vi "CRYGraph Octave Window.vi"() -> ()   [LabVIEW 2013]
uses:
  <vilib>/Utility/miscctls.llb/LVPoint32TypeDef.ctl
  Control/CRYFlag Cluster.ctl
  <vilib>/Utility/miscctls.llb/LVRowAndColumnTypeDef.ctl
  <vilib>/Utility/miscctls.llb/LVRectTypeDef.ctl
  SubVI/CRYData View Global.vi
  SubVI/CRYMain Sub Window Global.vi
  CRYCurveLibrary/Global/CRYCurve Library Global.vi
panel:
  out "LegendVScrollShow":bool=TRUE
  out "Legend Ref":refnum<vi>
  out "SelectedRow":i32[](array[numeric])
  in  "LoadFinish":bool
  in  "ScaleFitY 2":bool
  in  "ScaleFitY":bool
  in  "ScaleFitX":bool
  in  "ToolbarUpdate":bool
  out "PropertyTab":string
  in  "OpenProperty":bool
  in  "PaletteShow":bool
  in  "FitPanes":bool
  in  "DirectionKey":bool
  out "Graph Ref":refnum<vi>
  out "Repaint Watermark":i32
  out "Event Name":string
  out "ReportDrop":bool
  in  "AxisChange":bool
  in  "RemoveSome":bool
  in  "RemoveAll":bool
  in  "CursorColor":bool
  out "NewCursIdx":u32
  out "Test":string
  in  "OldCursIdx":u32
  out "Queue Name":string
  in  "StateOut":bool
  out "Cursor Coords":T1
  in  "CursorPlot":bool
  out "Cursor Ref":refnum<vi>
  in  "CursorShow":bool
  out "Octave Graph":cluster{"XY Graph":cluster{dbl, dbl}[]}[](graph)
  out "Title Name":string
  out "OldRow":i32
  out "TotalPlot":u32
  out "Graph Number":i32
  in  "stop":bool
  in  "CursorEnabled":bool
  in  "Cursor":string[][](table)
  in  "LegendShow":bool
  in  "ColorBox":u32(colorbox)
  in  "Legend":i32[](listbox)
  in  "GraphType":string
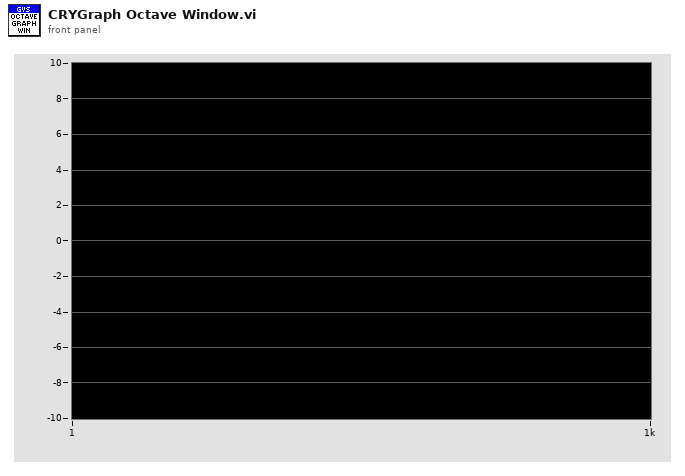
[diagram p1: front panel]
types:
  T1 = typedef "LVPoint32TypeDef.ctl" = cluster{"Horizontal":i32, "Vertical":i32}
  T2 = typedef "CRYFlag Cluster.ctl" = cluster{"LegendShow":bool, "CellClick":bool, "Total Number":bool, "ScaleFitX":bool, "ScaleFitY":bool, "MapModeX":u8, "MapModeY":u8, "CursorShow":bool, "MagnitudeShow":bool, "PreviewShow":bool, "CursorEnabled":bool, "IntensityShow":bool, "PaletteShow":bool, "PhaseShow":bool, "XYShow":bool, "FrequencyShow":bool, "LegendVScrollShow":bool, "FrequencyVScrollShow":bool}
  T3 = typedef "CRYGraph Event.ctl" = cluster{"EvenName":string, "TitleName":string, "GraphName":string, "GraphType":string, "Data":variant, "Queue Name":string, "DataView Number":i32}
  T4 = enum16{"No Scaling", "Scale All Objects", "Scale Single Object"}
  T5 = typedef "LVRowAndColumnTypeDef.ctl" = cluster{"Row":i32, "Column":i32}
  T6 = typedef "LVRectTypeDef.ctl" = cluster{"Left":i16, "Top":i16, "Right":i16, "Bottom":i16}
  T7 = typedef "LVBoundsTypeDef.ctl" = cluster{"Width":u32, "Height":u32}
  T8 = typedef "LVPositionTypeDef.ctl" = cluster{"Left":i32, "Top":i32}
  T9 = typedef "CRYData Cluster.ctl" = cluster{"Name":string, "Curve":cluster{"x":dbl, "y":dbl, "z":dbl}[], "X data":u16, "Y data":u16, "Z data":u16, "X axis":u16, "Y axis":u16, "Z axis":u16, "X unit":string, "Y unit":string, "Z unit":string, "X dB ref":dbl, "Y dB ref":dbl, "Z dB ref":dbl, "single val":bool, "protected":bool, "display X":bool, "display Y":bool, "display Z":bool, "Test Info":string, "Step No.":i32, "Plot Settings":cluster{"Color":u32, "Interpolation":u8, "Point Style":u8, "Line Style":u8, "Point Color":u32, "Line Width":u8, "Bar Plot Style":u8, "Fill To":i16}, "AutoProtect":bool}
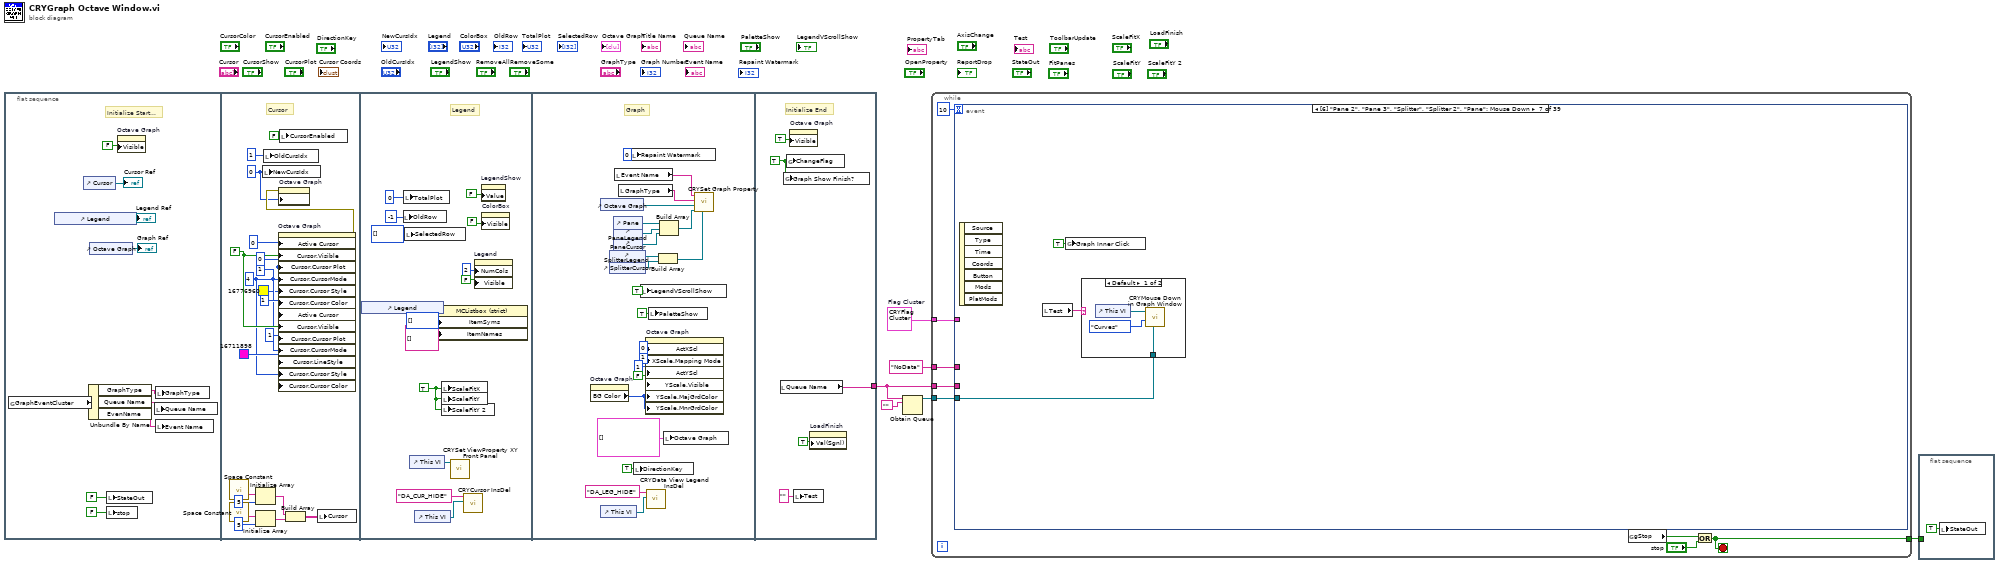
[diagram p0: block diagram]
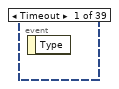
[diagram p2: hidden frame]
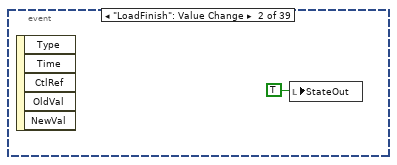
[diagram p3: hidden frame]
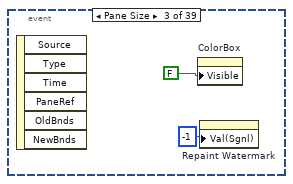
[diagram p4: hidden frame]
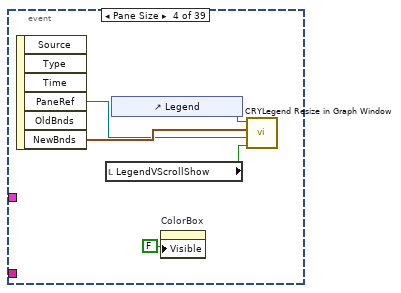
[diagram p5: hidden frame]
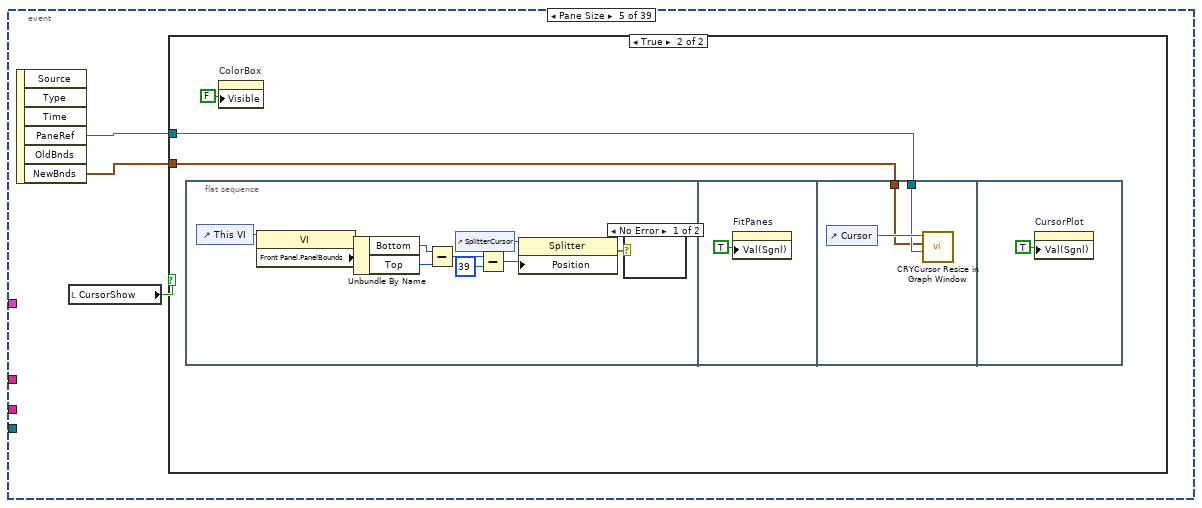
[diagram p6: hidden frame]
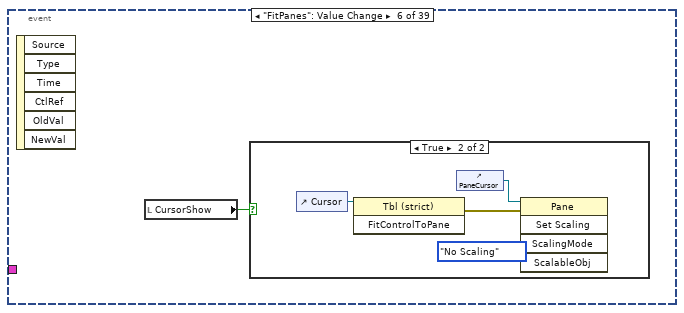
[diagram p9: hidden frame]
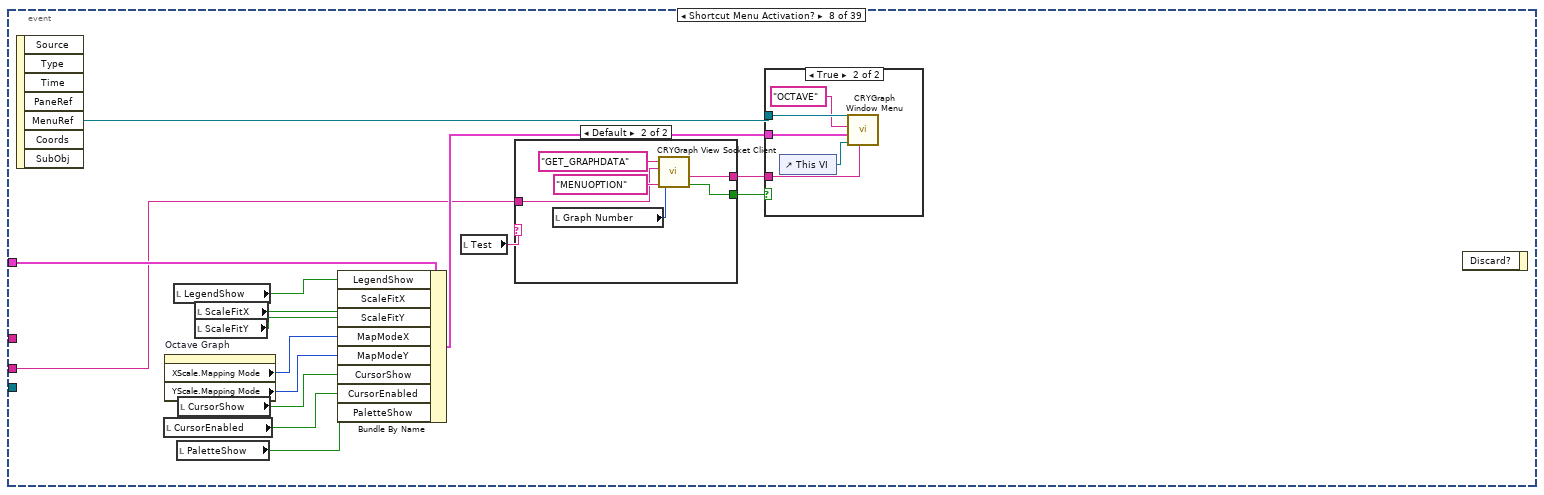
[diagram p12: hidden frame]
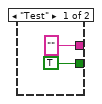
[diagram p13: hidden frame]
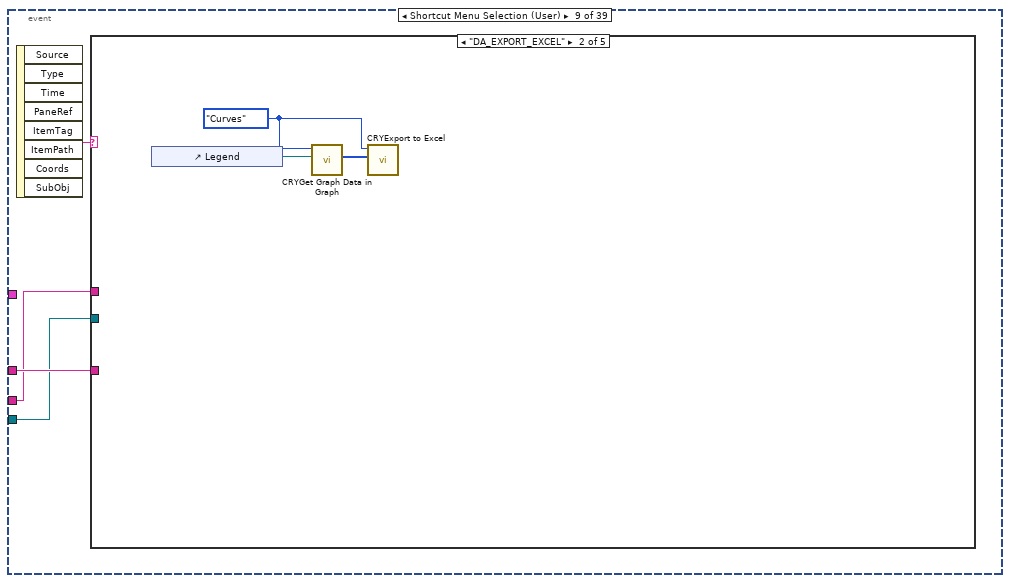
[diagram p15: hidden frame]
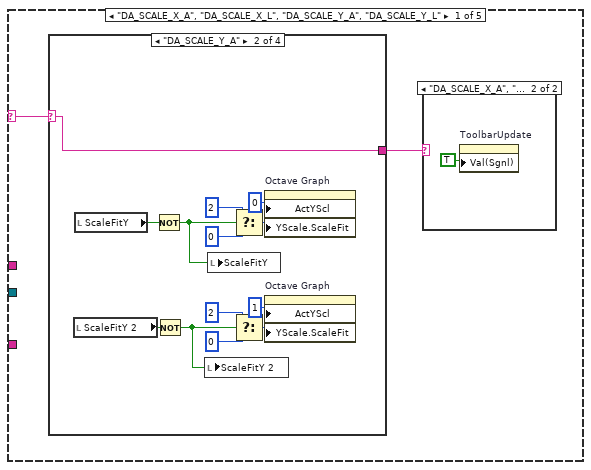
[diagram p16: hidden frame]
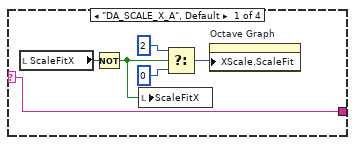
[diagram p18: hidden frame]
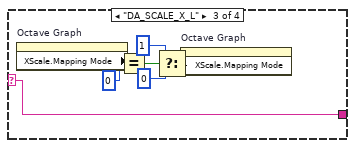
[diagram p19: hidden frame]
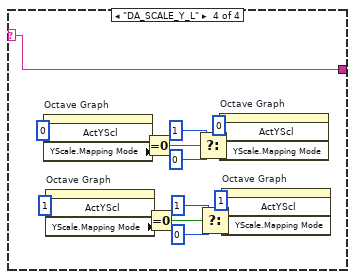
[diagram p20: hidden frame]
diagram:
  w4 = T2 {"LegendShow"=FALSE, "CellClick"=FALSE, "Total Number"=FALSE, "ScaleFitX"=FALSE, "ScaleFitY"=FALSE, "MapModeX"=0, "MapModeY"=0, "CursorShow"=FALSE, "MagnitudeShow"=FALSE, "PreviewShow"=FALSE, "CursorEnabled"=FALSE, "IntensityShow"=FALSE, "PaletteShow"=FALSE, "PhaseShow"=FALSE, "XYShow"=FALSE, "FrequencyShow"=FALSE, "LegendVScrollShow"=FALSE, "FrequencyVScrollShow"=FALSE}  # Flag Cluster
  n1 = flat-sequence {
    tunnel: [w74] -> w2
    frame #0 {
      # "Initialize Start..."
      n2 = global read "CRYData View Global.vi" "GraphEventCluster"() -> (w12:T3)
      n3 = control-ref of="Legend"() -> (→"Legend Ref":refnum<vi>)
      n4 = control-ref of="Cursor"() -> (→"Cursor Ref":refnum<vi>)
      n5 = Unbundle By Name(w12) -> ("GraphType"=w10:string, "Queue Name"=w11:string, "EvenName"=w9:string)
      n6 = control-ref of="Octave Graph"() -> (→"Graph Ref":refnum<vi>)
      n7 = local write "StateOut"(FALSE ("StateOut")) -> ()
      n8 = local write "stop"(FALSE ("stop")) -> ()
      n9 = property on="Octave Graph" class="XYGraph (strict)"("Visible"=FALSE) -> ()  [unwired: 2 in, 2 out]
      n10 = local write "Queue Name"(w11) -> ()
      n11 = local write "GraphType"(w10) -> ()
      n12 = local write "Event Name"(w9) -> ()
    }
    frame #1 {
      w22 = u32 0 ("Active Cursor")
      w17 = u8 4 ("Cursor.Cursor Style")
      w24 = u32 1 ("Cursor.Cursor Mode")
      w25 = 0 ("Cursor.Cursor Plot")
      w26 = FALSE ("Cursor.Visible")
      # "Cursor"
      n13 = call <vilib>:"Space Constant.vi"() -> ("String"=w30:string)
      n14 = call <vilib>:"Space Constant.vi"() -> ("String"=w35:string)
      n15 = Initialize Array(w30, 5 ("dimension size")) -> (w32:string[])
      n16 = Initialize Array(w35, 5 ("dimension size")) -> (w36:string[])
      n17 = local write "NewCursIdx"(w22) -> ()
      n18 = local write "OldCursIdx"(u32 1 ("OldCursIdx")) -> ()
      n19 = property on="Octave Graph" class="XYGraph (strict)"("Active Cursor"=u32 0, "Cursor.Visible"=w26, "Cursor.Cursor Plot"=w25, "Cursor.CursorMode"=w24, "Cursor.Cursor Style"=w17, "Cursor.Cursor Color"=u32 16776960, "Active Cursor"=u32 1, "Cursor.Visible"=w26, "Cursor.Cursor Plot"=w25, "Cursor.CursorMode"=w24, "Cursor.LineStyle"=u8 1 ("Cursor.Line Style"), "Cursor.Cursor Style"=w17, "Cursor.Cursor Color"=u32 16711898) -> (error out=w23:errorcluster)  [unwired: 2 in, 1 out]
      n20 = property on="Octave Graph" class="XYGraph (strict)"(error in=w23, "Active Cursor"=w22) -> ()  [unwired: 1 in, 2 out]
      n21 = local write "CursorEnabled"(FALSE ("CursorEnabled")) -> ()
      n22 = Build Array(w32, w36) -> (w33:string[][])
      n23 = local write "Cursor"(w33) -> ()
    }
    frame #2 {
      w38 = TRUE ("ScaleFitX")
      # "Legend"
      n24 = control-ref of="Legend"() -> (w50:refnum<vi>)
      n25 = local write "OldRow"(-1 ("OldRow 2")) -> ()
      n26 = local write "TotalPlot"(u32 0 ("TotalPlot")) -> ()
      n27 = local write "SelectedRow"(i32[] [] ("SelectedRow")) -> ()
      n28 = control-ref of="This VI"() -> (w39:refnum<vi>)
      n29 = control-ref of="This VI"() -> (w41:refnum<vi>)
      n30 = property on="Property Node" class="MCListbox (strict)"(reference=w50, "ItemSyms"=i32[] [] ("Item Symbols"), "ItemNames"=string[][] [] ("Item Names")) -> ()  [unwired: 1 in, 2 out]
      n31 = local write "ScaleFitX"(w38) -> ()
      n32 = local write "ScaleFitY"(w38) -> ()
      n33 = local write "ScaleFitY 2"(w38) -> ()
      n34 = call "CRYSet ViewProperty XY  Front Panel.vi"("Vi Ref"=w39) -> ()  [unwired: 11 in]
      n35 = call "CRYCursor InsDel.vi"("Graph VI Ref"=w41, "sAction"="DA_CUR_HIDE" ("Action Type")) -> ()  [unwired: 10 in]
      n36 = property on="Legend" class="MCListbox (strict)"("NumCols"=u32 2 ("Number of Columns"), "Visible"=FALSE) -> ()  [unwired: 2 in, 2 out]
      n37 = property on="LegendShow" class="Bool (strict)"("Value"=FALSE ("Visible")) -> ()  [unwired: 2 in, 2 out]
      n38 = property on="ColorBox" class="ColBox"("Visible"=FALSE) -> ()  [unwired: 2 in, 2 out]
    }
    frame #3 {
      # "Graph"
      n39 = property on="Octave Graph" class="XYGraph (strict)"() -> ("BG Color"=w70:u32)  [unwired: 2 in, 2 out]
      n40 = control-ref of="Octave Graph"() -> (w60:refnum<vi>)
      n41 = control-ref of="This VI"() -> (w52:refnum<vi>)
      n42 = control-ref of="SplitterLegend"() -> (w69:refnum<vi>)
      n43 = control-ref of="SplitterCursor"() -> (w68:refnum<vi>)
      n44 = control-ref of="Pane"() -> (w66:refnum<vi>)
      n45 = control-ref of="PaneLegend"() -> (w67:refnum<vi>)
      n46 = control-ref of="PaneCursor"() -> (w55:refnum<vi>)
      n47 = local read "Event Name"() -> (w62:string)
      n48 = local read "GraphType"() -> (w63:string)
      n49 = local write "Repaint Watermark"(0 ("Repaint Watermark")) -> ()
      n50 = local write "DirectionKey"(TRUE ("DirectionKey")) -> ()
      n51 = local write "LegendVScrollShow"(TRUE ("LegendVScrollShow")) -> ()
      n52 = property on="Octave Graph" class="XYGraph (strict)"("ActXScl"=0 ("Active X Scale"), "XScale.Mapping Mode"=u8 1 ("X Scale.Mapping Mode"), "ActYScl"=1 ("Active Y Scale"), "YScale.Visible"=FALSE ("Y Scale.Visible"), "YScale.MajGrdColor"=w70, "YScale.MnrGrdColor"=w70) -> ()  [unwired: 2 in, 2 out]
      n53 = call "CRYData View Legend InsDel.vi"("Graph VI Ref"=w52, "sAction"="DA_LEG_HIDE" ("Action Type")) -> ()  [unwired: 2 in, 8 out]
      n54 = local write "PaletteShow"(TRUE ("PaletteShow")) -> ()
      n55 = Build Array(w69, w68) -> (w64:refnum<vi>[])
      n56 = Build Array(w66, w67, w55) -> (w65:refnum<vi>[])
      n57 = local write "Octave Graph"(cluster{"XY Graph":cluster{dbl, dbl}[]}[] [] ("XY Graph")) -> ()
      n58 = call "CRYSet Graph Property.vi"("Splitters"=w64, "Panes"=w65, "Graph Ref"=w60, "Graph Type"=w63, "Event Name"=w62) -> ()  [unwired: 7 in]
    }
    frame #4 {
      w77 = TRUE ("ChangeFlag")
      # "Initialize End"
      n59 = local read "Queue Name"() -> (w74:string)
      n60 = global write "CRYData View Global.vi" "Graph Show Finish?"(w77) -> ()
      n61 = global write "CRYData View Global.vi" "ChangeFlag"(w77) -> ()
      n62 = property on="Octave Graph" class="XYGraph (strict)"("Visible"=TRUE) -> ()  [unwired: 2 in, 2 out]
      n63 = local write "Test"("" ("Test")) -> ()
      n64 = property on="LoadFinish" class="Bool (strict)"("Val(Sgnl)"=TRUE ("Value (Signaling)")) -> ()  [unwired: 2 in, 2 out]
    }
  }
  n65 = Obtain Queue(name (unnamed)=w2, element data type="") -> (queue out=w6:refnum<queue>)  [unwired: 3 in, 2 out]
  n66 = while {
    tunnel: w6 -> [w85]
    tunnel: w4 -> [w83]
    tunnel: "NoData" ("input 2") -> [w80]
    tunnel: w2 -> [w79]
    tunnel: [w78] -> w1
    stop <- w78 stop-if-true
    n67 = event shown="[6] \"Pane 2\", \"Pane 3\", \"Splitter\", \"Splitter 2\", \"Pane\": Mouse Down" {
      selector: _ -> [_ _ _ _ _ _ _ _ _ _ _ _ _ _ _ _ _ _ _ _ _ _ _ _ _ _ _ _ _ _ _ _ _ _ _ _ _ _ _]
      dyn-events: _ -> [_ _ _ _ _ _ _ _ _ _ _ _ _ _ _ _ _ _ _ _ _ _ _ _ _ _ _ _ _ _ _ _ _ _ _ _ _ _ _]
      timeout: 10 -> [_ _ _ _ _ _ _ _ _ _ _ _ _ _ _ _ _ _ _ _ _ _ _ _ _ _ _ _ _ _ _ _ _ _ _ _ _ _ _]
      tunnel: w85 -> [_ _ _ _ _ _ w121 _ w153 _ w265 _ w318 _ _ _ _ _ _ _ _ _ _ _ _ w525 _ _ _ _ _ w731 _ _ w743 _ _ _ _]
      tunnel: w83 -> [_ _ _ _ _ _ _ w137 _ w242 _ w303 _ _ _ _ _ _ _ _ _ _ _ _ _ _ _ _ _ _ _ _ _ _ _ _ _ _ _]
      tunnel: w80 -> [_ _ _ _ _ _ _ _ w155 _ w262 _ w317 _ _ _ _ _ _ _ _ _ _ _ _ _ _ _ _ _ _ _ _ _ _ _ _ _ _]
      tunnel: w79 -> [_ _ _ _ _ _ _ w131 w154 _ _ _ _ _ _ _ _ _ _ _ _ _ _ _ _ _ _ _ _ _ _ _ _ _ _ _ _ _ _]
      event Timeout {
        n68 = event-data() -> ()  [unwired: 2 out]
      }
      event "LoadFinish": Value Change {
        n69 = event-data() -> ()  [unwired: 6 out]
        n70 = local write "StateOut"(TRUE ("StateOut")) -> ()
      }
      event Pane Size {
        n71 = event-data() -> ()  [unwired: 7 out]
        n72 = property on="ColorBox" class="ColBox"("Visible"=FALSE) -> ()  [unwired: 2 in, 2 out]
        n73 = property on="Repaint Watermark" class="DigNum (strict)"("Val(Sgnl)"=-1 ("Value (Signaling)")) -> ()  [unwired: 2 in, 2 out]
      }
      event Pane Size {
        n74 = event-data() -> ("PaneRef"=w90:refnum<vi>, "NewBnds"=w92:T6)  [unwired: 5 out]
        n75 = local read "LegendVScrollShow"() -> (w89:bool)
        n76 = control-ref of="Legend"() -> (w91:refnum<vi>)
        n77 = property on="ColorBox" class="ColBox"("Visible"=FALSE) -> ()  [unwired: 2 in, 2 out]
        n78 = call "CRYLegend Resize in Graph Window.vi"("VScrollShow"=w89, "Pane Ref"=w90, "input cluster"=w92, "Legend"=w91) -> ()  [unwired: 8 out]
      }
      event Pane Size {
        n79 = event-data() -> ("PaneRef"=w95:refnum<vi>, "NewBnds"=w94:T6)  [unwired: 5 out]
        n80 = local read "CursorShow"() -> (w96:bool)
        n81 = case shown="True" w96 {
          tunnel: w95 -> [_ w98]
          tunnel: w94 -> [_ w97]
          frame False {
          }
          frame True {
            n82 = flat-sequence {
              tunnel: w98 -> [w111]
              tunnel: w97 -> [w110]
              frame #0 {
                n83 = control-ref of="This VI"() -> (w103:refnum<vi>)
                n84 = property class="VI"(reference=w103) -> ("Front Panel.PanelBounds"=w104:T6)  [unwired: 1 in, 2 out]
                n85 = Unbundle By Name(w104) -> ("Bottom"=w101:i16, "Top"=w102:i16)
                n86 = Subtract(x=w101, y=w102) -> (x-y=w105:i16)
                n87 = control-ref of="SplitterCursor"() -> (w108:refnum<vi>)
                n88 = Subtract(x=w105, y=39) -> (x-y=w100:i32)
                n89 = property class="Splitter"(reference=w108, "Position"=w100) -> (error out=w107:errorcluster)  [unwired: 1 in, 1 out]
                n90 = case shown="No Error" w107 {
                  frame No Error {
                  }
                  frame Error {
                  }
                }
              }
              frame #1 {
                n91 = property on="FitPanes" class="Bool (strict)"("Val(Sgnl)"=TRUE ("Value (Signaling)")) -> ()  [unwired: 2 in, 2 out]
              }
              frame #2 {
                n92 = control-ref of="Cursor"() -> (w112:refnum<vi>)
                n93 = call "CRYCursor Resize in Graph Window.vi"("Pane Ref"=w111, "input cluster"=w110, "Graph Cursor Ref"=w112) -> ()  [unwired: 9 in]
              }
              frame #3 {
                n94 = property on="CursorPlot" class="Bool (strict)"("Val(Sgnl)"=TRUE ("Value (Signaling)")) -> ()  [unwired: 2 in, 2 out]
              }
            }
            n95 = property on="ColorBox" class="ColBox"("Visible"=FALSE) -> ()  [unwired: 2 in, 2 out]
          }
        }
      }
      event "FitPanes": Value Change {
        n96 = event-data() -> ()  [unwired: 7 out]
        n97 = local read "CursorShow"() -> (w114:bool)
        n98 = case shown="True" w114 {
          frame False {
          }
          frame True {
            n99 = control-ref of="Cursor"() -> (w118:refnum<vi>)
            n100 = invoke class="Tbl (strict)" method="FitControlToPane"(reference=w118) -> (error out=w117:errorcluster)  [unwired: 2 in, 2 out]
            n101 = control-ref of="PaneCursor"() -> (w115:refnum<vi>)
            n102 = invoke class="Pane" method="Set Scaling"(reference=w115, error in=w117, "ScalingMode"=T4."No Scaling" ("Scaling Mode")) -> ()  [unwired: 2 in, 5 out]
          }
        }
      }
      event Mouse Down {
        n103 = event-data() -> ()  [unwired: 8 out]
        n104 = local read "Test"() -> (w120:string)
        n105 = global write "CRYCurve Library Global.vi" "Graph Inner Click"(TRUE ("Graph Inner Click")) -> ()
        n106 = case shown="Default" w120 {
          tunnel: w121 -> [w124 _]
          frame Default {
            n107 = control-ref of="This VI"() -> (w122:refnum<vi>)
            n108 = call "CRYMouse Down in Graph Window.vi"("Queue"=w124, "Selected Type"=enum16{"Curves", "Values", "Results", "WFM"}."Curves" ("Type"), "pGraph VI In"=w122) -> ()  [unwired: 3 in, 6 out]
          }
          frame "Test" {
          }
        }
      }
      event Shortcut Menu Activation? {
        n109 = event-data() -> ("MenuRef"=w139:refnum<k9>)  [unwired: 7 out]
        n110 = local read "CursorEnabled"() -> (w132:bool)
        n111 = property on="Octave Graph" class="XYGraph (strict)"() -> ("XScale.Mapping Mode"=w135:u8, "YScale.Mapping Mode"=w134:u8)  [unwired: 2 in, 2 out]
        n112 = local read "LegendShow"() -> (w138:bool)
        n113 = local read "PaletteShow"() -> (w127:bool)
        n114 = local read "CursorShow"() -> (w133:bool)
        n115 = local read "ScaleFitX"() -> (w126:bool)
        n116 = local read "ScaleFitY"() -> (w125:bool)
        n117 = Bundle By Name(cluster=w137, "LegendShow"=w138, "ScaleFitX"=w126, "ScaleFitY"=w125, "MapModeX"=w135, "MapModeY"=w134, "CursorShow"=w133, "CursorEnabled"=w132, "PaletteShow"=w127) -> (w136:T2)
        n118 = local read "Test"() -> (w128:string)
        n119 = case shown="Default" w128 {
          tunnel: w131 -> [_ w145]
          tunnel: ["" ("sData Out") w144] -> w130
          tunnel: [TRUE ("bResult Out") w143] -> w129
          frame "Test" {
          }
          frame Default {
            n120 = local read "Graph Number"() -> (w142:i32)
            n121 = call "CRYGraph View Socket Client.vi"("sOption"="MENUOPTION", "nData"=w142, "sData"=w145, "sAction"="GET_GRAPHDATA") -> ("bResult Out"=w143:bool, "sData Out"=w144:string)  [unwired: 4 in, 2 out]
          }
        }
        n122 = case shown="True" w129 {
          tunnel: w139 -> [_ w152]
          tunnel: w136 -> [_ w150]
          tunnel: w130 -> [_ w149]
          frame False {
          }
          frame True {
            n123 = control-ref of="This VI"() -> (w148:refnum<vi>)
            n124 = call "CRYGraph Window Menu.vi"("MenuOption"=w149, "pGraph VI"=w148, "Flag Cluster"=w150, "Type"="OCTAVE", "Runtime Menu Ref In"=w152) -> ()  [unwired: 7 out]
          }
        }
        n125 = event-data() -> ()  [unwired: 2 in, 1 out]
      }
      event Shortcut Menu Selection (User) {
        n126 = event-data() -> ("ItemTag"=w156:string)  [unwired: 8 out]
        n127 = case shown="\"DA_EXPORT_EXCEL\"" w156 {
          selector: w156 -> [w158 _ w205 w238 _]
          tunnel: w155 -> [_ _ w208 _ _]
          tunnel: w154 -> [_ _ _ _ _]
          tunnel: w153 -> [_ _ w206 _ _]
          frame "DA_SCALE_X_A", "DA_SCALE_X_L", "DA_SCALE_Y_A", "DA_SCALE_Y_L" {
            n128 = case shown="\"DA_SCALE_Y_A\"" w158 {
              selector: w158 -> [w162 w175 w179 w200]
              tunnel: [w162 w175 w179 w200] -> w157
              frame "DA_SCALE_X_A", Default {
                n129 = local read "ScaleFitX"() -> (w161:bool)
                n130 = Not(x=w161) -> (.not. x?=w160:bool)
                n131 = local write "ScaleFitX"(w160) -> ()
                n132 = Select(t=u8 2, s=w160, f=u8 0) -> (s? t:f=w163:u8)
                n133 = property on="Octave Graph" class="XYGraph (strict)"("XScale.ScaleFit"=w163) -> ()  [unwired: 2 in, 2 out]
              }
              frame "DA_SCALE_Y_A" {
                n134 = local read "ScaleFitY 2"() -> (w168:bool)
                n135 = local read "ScaleFitY"() -> (w169:bool)
                n136 = Not(x=w169) -> (.not. x?=w167:bool)
                n137 = Not(x=w168) -> (.not. x?=w166:bool)
                n138 = local write "ScaleFitY 2"(w166) -> ()
                n139 = local write "ScaleFitY"(w167) -> ()
                n140 = Select(t=u8 2, s=w167, f=u8 0) -> (s? t:f=w176:u8)
                n141 = Select(t=u8 2, s=w166, f=u8 0) -> (s? t:f=w172:u8)
                n142 = property on="Octave Graph" class="XYGraph (strict)"("ActYScl"=0 ("Active Y Scale"), "YScale.ScaleFit"=w176) -> ()  [unwired: 2 in, 2 out]
                n143 = property on="Octave Graph" class="XYGraph (strict)"("ActYScl"=1 ("Active Y Scale"), "YScale.ScaleFit"=w172) -> ()  [unwired: 2 in, 2 out]
              }
              frame "DA_SCALE_X_L" {
                n144 = property on="Octave Graph" class="XYGraph (strict)"() -> ("XScale.Mapping Mode"=w180:u8)  [unwired: 2 in, 2 out]
                n145 = Equal?(x=w180, y=u8 0) -> (x = y?=w185:bool)
                n146 = Select(t=u8 1, s=w185, f=u8 0) -> (s? t:f=w181:u8)
                n147 = property on="Octave Graph" class="XYGraph (strict)"("XScale.Mapping Mode"=w181) -> ()  [unwired: 2 in, 2 out]
              }
              frame "DA_SCALE_Y_L" {
                n148 = property on="Octave Graph" class="XYGraph (strict)"("ActYScl"=0 ("Active Y Scale")) -> ("YScale.Mapping Mode"=w196:u8)  [unwired: 2 in, 2 out]
                n149 = property on="Octave Graph" class="XYGraph (strict)"("ActYScl"=1 ("Active Y Scale")) -> ("YScale.Mapping Mode"=w189:u8)  [unwired: 2 in, 2 out]
                n150 = Equal To 0?(x=w196) -> (x = 0?=w193:bool)
                n151 = Equal To 0?(x=w189) -> (x = 0?=w192:bool)
                n152 = Select(t=u8 1, s=w193, f=u8 0) -> (s? t:f=w197:u8)
                n153 = Select(t=u8 1, s=w192, f=u8 0) -> (s? t:f=w188:u8)
                n154 = property on="Octave Graph" class="XYGraph (strict)"("ActYScl"=0 ("Active Y Scale"), "YScale.Mapping Mode"=w197) -> ()  [unwired: 2 in, 2 out]
                n155 = property on="Octave Graph" class="XYGraph (strict)"("ActYScl"=1 ("Active Y Scale"), "YScale.Mapping Mode"=w188) -> ()  [unwired: 2 in, 2 out]
              }
            }
            n156 = case shown="\"DA_SCALE_X_A\", \"DA_SCALE_Y_A\"" w157 {
              frame Default {
              }
              frame "DA_SCALE_X_A", "DA_SCALE_Y_A" {
                n157 = property on="ToolbarUpdate" class="Bool (strict)"("Val(Sgnl)"=TRUE ("Value (Signaling)")) -> ()  [unwired: 2 in, 2 out]
              }
            }
          }
          frame "DA_EXPORT_EXCEL" {
            w202 = enum16{"Curves", "Values", "Results", "WFM"}."Curves" ("Type")
            n158 = control-ref of="Legend"() -> (w201:refnum<vi>)
            n159 = call "CRYGet Graph Data in Graph.vi"("Legend Refnum"=w201, "Type In"=w202) -> ("Rows"=w203:i32[])  [unwired: 2 in, 7 out]
            n160 = call "CRYExport to Excel.vi"("Rows"=w203, "Type"=w202) -> ()  [unwired: 2 in, 8 out]
          }
          frame Default {
            n161 = Search/Split String(string=w205, search string/char (-)="#") -> (substring before match=w204:string, match + rest of string=w211:string)  [unwired: 2 out]
            n162 = call "CRYPreUpdate Sequence.vi"("EventName"="CurLibUpdate") -> ()  [unwired: 15 in]
            n163 = Decimal String To Number(string=w211, offset=1) -> (number=w209:i32)  [unwired: 2 out]
            n164 = case shown="0, Default" w209 {
              selector: w209 -> [_ w225]
              tunnel: w204 -> [w215 w227]
              tunnel: w208 -> [_ _]
              tunnel: w206 -> [w219 w223]
              frame 0, Default {
                n165 = local read "GraphType"() -> (w213:string)
                n166 = local read "Graph Number"() -> (w220:i32)
                n167 = Equal?(x="DA_EXPORT_DOCUMENT" ("y"), y=w215) -> (x = y?=w218:bool)
                n168 = Select(t="ADD_DOC", s=w218, f=w215) -> (s? t:f=w214:string)
                n169 = Format Into String(w214, w213, w220, 0 ("input 3")) -> (resulting string=w221:string)  [unwired: 3 in, 1 out]
                n170 = Enqueue Element(queue=w219, element=w221) -> ()  [unwired: 1 in, 4 out]
              }
              frame 1..10 {
                n171 = flat-sequence {
                  tunnel: w227 -> [w230]
                  tunnel: [w230] -> w226
                  tunnel: w225 -> [w229]
                  tunnel: [w228] -> w224
                  tunnel: w226 -> [w234]
                  tunnel: w224 -> [w232]
                  tunnel: w223 -> [w231]
                  frame #0 {
                    n172 = call "CRYSet Graph Cluster Data.vi"("Graph Number"=w229) -> ("DataType"=w228:string)  [unwired: 2 in, 8 out]
                  }
                  frame #1 {
                    n173 = local read "Graph Number"() -> (w233:i32)
                    n174 = Format Into String(w234, w232, w233, 0 ("input 3")) -> (resulting string=w236:string)  [unwired: 3 in, 1 out]
                    n175 = Enqueue Element(queue=w231, element=w236) -> ()  [unwired: 1 in, 4 out]
                  }
                }
              }
            }
          }
          frame "DA_PAL_HIDE", "DA_PAL_VIEW" {
            n176 = Equal?(x=w238, y="DA_PAL_VIEW") -> (x = y?=w237:bool)
            n177 = property on="PaletteShow" class="Bool (strict)"("Val(Sgnl)"=w237) -> ()  [unwired: 2 in, 2 out]
          }
          frame "DA_REMOVEALL" {
            n178 = property on="RemoveAll" class="Bool (strict)"("Val(Sgnl)"=TRUE ("Value (Signaling)")) -> ()  [unwired: 2 in, 2 out]
          }
        }
      }
      event Shortcut Menu Activation? {
        n179 = event-data() -> ("MenuRef"=w243:refnum<k9>, "Coords"=w244:T1)  [unwired: 6 out]
        n180 = local read "LegendShow"() -> (w241:bool)
        n181 = case shown="True" w241 {
          selector: w241 -> [_ w249]
          tunnel: w244 -> [_ w260]
          tunnel: w243 -> [_ w258]
          tunnel: w242 -> [_ w254]
          frame False {
          }
          frame True {
            n182 = invoke on="Legend" class="MCListbox (strict)" method="Point To Row Column"("Point"=w260) -> ("CellPosition"=w261:T5)  [unwired: 6 in, 6 out]
            n183 = local read "TotalPlot"() -> (w252:u32)
            n184 = control-ref of="Legend"() -> (w248:refnum<vi>)
            n185 = Unbundle By Name(w261) -> ("Row"=w246:i32)
            n186 = To Long Integer(number=w252) -> (32bit integer=w251:i32)
            n187 = local read "LegendVScrollShow"() -> (w245:bool)
            n188 = Less?(x=w246, y=w251) -> (x < y?=w256:bool)
            n189 = local write "OldRow"(w246) -> ()
            n190 = Greater?(x=w252, y=u32 0) -> (0:w255:bool)
            n191 = call "CRYGet Selected Data in Legend.vi"("Right Clicked Row"=w246, "Legend Ref"=w248) -> ("Selected Rows"=w247:i32[])  [unwired: 9 in]
            n192 = local write "SelectedRow"(w247) -> ()
            n193 = property on="Legend" class="MCListbox (strict)"("Value"=w247) -> ()  [unwired: 2 in, 2 out]
            n194 = Bundle By Name(cluster=w254, "LegendShow"=w249, "CellClick"=w256, "Total Number"=w255, "LegendVScrollShow"=w245) -> (w253:T2)
            n195 = control-ref of="This VI"() -> (w250:refnum<vi>)
            n196 = call "CRYGraph Window Menu.vi"("pGraph VI"=w250, "Flag Cluster"=w253, "Type"="LEGEND", "Runtime Menu Ref In"=w258) -> ()  [unwired: 1 in, 7 out]
          }
        }
        n197 = event-data() -> ()  [unwired: 1 in, 2 out]
      }
      event Shortcut Menu Selection (User) {
        n198 = event-data() -> ("ItemTag"=w266:string)  [unwired: 8 out]
        n199 = local read "Graph Number"() -> (w263:i32)
        n200 = case shown="\"DA_LEG_VSCROLL_HIDE\", \"DA_LEG_VSCROLL_VIEW\"" w266 {
          selector: w266 -> [_ _ _ _ _ _ w300]
          tunnel: w265 -> [_ w271 _ _ _ _ _]
          tunnel: w263 -> [_ w270 _ _ _ _ _]
          tunnel: w262 -> [_ w268 _ _ _ _ _]
          frame Default {
          }
          frame "DA_LEG_HIDE_1" {
            n201 = Format Into String("DA_LEG_HIDE" ("input 2"), w268, w270, 0 ("input 3")) -> (resulting string=w272:string)  [unwired: 3 in, 1 out]
            n202 = Enqueue Element(queue=w271, element=w272) -> ()  [unwired: 1 in, 4 out]
          }
          frame "DA_LEG_REMOVE" {
            n203 = property on="RemoveSome" class="Bool (strict)"("Val(Sgnl)"=TRUE ("Value (Signaling)")) -> ()  [unwired: 2 in, 2 out]
          }
          frame "DA_LEG_REMOVEALL" {
            n204 = property on="RemoveAll" class="Bool (strict)"("Val(Sgnl)"=TRUE ("Value (Signaling)")) -> ()  [unwired: 2 in, 2 out]
          }
          frame "DA_LEG_INVERT" {
            n205 = local read "TotalPlot"() -> (w276:u32)
            n206 = for {
              N: w276 -> [_]
              tunnel: [w280] -> w277
              tunnel: [w279] -> w275
              i -> [w282]
              w284 = 38
              w286 = 37
              n207 = property on="Legend" class="MCListbox (strict)"() -> ("ItemSyms"=w288:i32[])  [unwired: 2 in, 2 out]
              n208 = Index Array(array=w288, index=w282) -> (element=w287:i32)
              n209 = To Unsigned Long Integer(number=w282) -> (unsigned 32bit integer=w281:u32)
              n210 = Equal?(x=w287, y=w286) -> (x = y?=w283:bool)
              n211 = Equal?(x=w287, y=w284) -> (x = y?=w285:bool)
              n212 = Select(t=w286, s=w285, f=w284) -> (s? t:f=w289:i32)
              n213 = Replace Array Subset(array=w288, new element=w289, index=w282) -> (w290:i32[])
              n214 = property on="Octave Graph" class="XYGraph (strict)"("Active Plot"=w281, "Plot.Visible?"=w283) -> (error out=w279:errorcluster)  [unwired: 2 in, 1 out]
              n215 = property on="Legend" class="MCListbox (strict)"("ItemSyms"=w290) -> (error out=w280:errorcluster)  [unwired: 2 in, 1 out]
            }
            n216 = case shown="No Error" w275 {
              frame No Error {
              }
              frame Error {
              }
            }
            n217 = property on="AxisChange" class="Bool (strict)"(error in=w277, "Val(Sgnl)"=TRUE ("Value (Signaling)")) -> ()  [unwired: 1 in, 2 out]
          }
          frame "DA_LEG_SHOWALL" {
            n218 = local read "TotalPlot"() -> (w291:u32)
            n219 = for {
              N: w291 -> [_]
              tunnel: [38] -> w294 mode=indexing
              i -> [w298]
              n220 = To Unsigned Long Integer(number=w298) -> (unsigned 32bit integer=w297:u32)
              n221 = property on="Octave Graph" class="XYGraph (strict)"("Active Plot"=w297, "Plot.Visible?"=TRUE ("Plot.Visible")) -> ()  [unwired: 2 in, 2 out]
            }
            n222 = property on="Legend" class="MCListbox (strict)"("ItemSyms"=w294) -> (error out=w293:errorcluster)  [unwired: 2 in, 1 out]
            n223 = property on="AxisChange" class="Bool (strict)"(error in=w293, "Val(Sgnl)"=TRUE ("Value (Signaling)")) -> ()  [unwired: 1 in, 2 out]
          }
          frame "DA_LEG_VSCROLL_HIDE", "DA_LEG_VSCROLL_VIEW" {
            n224 = Equal?(x="DA_LEG_VSCROLL_VIEW" ("y"), y=w300) -> (x = y?=w299:bool)
            n225 = property on="LegendVScrollShow" class="Bool (strict)"("Val(Sgnl)"=w299) -> ()  [unwired: 2 in, 2 out]
          }
        }
        n226 = call "CRYPreUpdate Sequence.vi"("EventName"="CurLibUpdate") -> ()  [unwired: 15 in]
      }
      event Shortcut Menu Activation? {
        n227 = event-data() -> ("MenuRef"=w304:refnum<k9>)  [unwired: 7 out]
        n228 = local read "CursorShow"() -> (w302:bool)
        n229 = case shown="True" w302 {
          selector: w302 -> [_ w305]
          tunnel: w304 -> [_ w308]
          tunnel: w303 -> [_ w307]
          frame False {
          }
          frame True {
            n230 = Bundle By Name(cluster=w307, "CursorShow"=w305) -> (w309:T2)
            n231 = control-ref of="This VI"() -> (w306:refnum<vi>)
            n232 = call "CRYGraph Window Menu.vi"("pGraph VI"=w306, "Flag Cluster"=w309, "Type"="CURSOR", "Runtime Menu Ref In"=w308) -> ()  [unwired: 1 in, 7 out]
          }
        }
        n233 = event-data() -> ()  [unwired: 2 in, 1 out]
      }
      event Shortcut Menu Selection (User) {
        n234 = event-data() -> ("ItemTag"=w313:string)  [unwired: 8 out]
        n235 = local read "Graph Number"() -> (w315:i32)
        n236 = Match Pattern(string=w313, regular expression="#" ("search string/char (-)")) -> (before substring=w312:string, after substring=w311:string)  [unwired: 1 in, 2 out]
        n237 = case shown="\"LINKTO\"" w312 {
          selector: w312 -> [_ _ _ w350 _]
          tunnel: w318 -> [_ _ _ w348 w355]
          tunnel: w315 -> [_ _ _ w351 w357]
          tunnel: w317 -> [_ _ _ w349 w356]
          tunnel: w311 -> [w319 _ w334 _ _]
          frame "DA_CUR_GOTO_CUR" {
            n238 = Decimal String To Number(string=w319) -> (number=w320:i32)  [unwired: 1 in, 2 out]
            n239 = case shown="0, 1" w320 {
              selector: w320 -> [_ w322]
              frame Default {
              }
              frame 0, 1 {
                n240 = flat-sequence {
                  tunnel: w322 -> [w324]
                  frame #0 {
                    n241 = Equal To 0?(x=w324) -> (x = 0?=w328:bool)
                    n242 = local write "NewCursIdx"(w324) -> ()
                    n243 = property on="Octave Graph" class="XYGraph (strict)"("Active Cursor"=w324) -> ()  [unwired: 2 in, 2 out]
                    n244 = Select(t=1 ("OldCursIdx"), s=w328, f=0 ("OldCursIdx")) -> (s? t:f=w325:i32)
                    n245 = local write "OldCursIdx"(w325) -> ()
                  }
                  frame #1 {
                    n246 = property on="CursorColor" class="Bool (strict)"("Val(Sgnl)"=TRUE ("Value (Signaling)")) -> ()  [unwired: 2 in, 2 out]
                  }
                }
                n247 = control-ref of="Octave Graph"() -> (w321:refnum<vi>)
                n248 = call "CRYGoto Cursor.vi"("Active Cursor"=w322, "Graph Ref"=w321, "Graph Type"="OCTAVE") -> ()  [unwired: 9 in]
              }
            }
          }
          frame "DA_BRING_CENTER" {
            n249 = property on="Octave Graph" class="XYGraph (strict)"() -> ("Active Cursor"=w331:u32)  [unwired: 2 in, 2 out]
            n250 = control-ref of="Octave Graph"() -> (w332:refnum<vi>)
            n251 = call "CRYGoto Cursor.vi"("sOption"="Bring_to_Center", "Active Cursor"=w331, "Graph Ref"=w332, "Graph Type"="OCTAVE") -> ()  [unwired: 8 in]
          }
          frame "LINKTO" {
            n252 = Match Pattern(string=w334, regular expression="[0-1]_") -> (match substring=w338:string, after substring=w336:string)  [unwired: 1 in, 2 out]
            n253 = Decimal String To Number(string=w338) -> (number=w335:i32)  [unwired: 2 in, 1 out]
            n254 = case shown="0, 1" w335 {
              selector: w335 -> [w339 _]
              tunnel: w336 -> [w340 _]
              frame 0, 1 {
                n255 = control-ref of="Legend"() -> (w342:refnum<vi>)
                n256 = call "CRYGet Legend Name.vi"("MCListbox Refnum"=w342) -> ("Names Out"=w343:string[])  [unwired: 10 in]
                n257 = control-ref of="Octave Graph"() -> (w341:refnum<vi>)
                n258 = Search 1D Array(1D array=w343, element=w340) -> (index of element=w344:i32)  [unwired: 1 in]
                n259 = case shown="0, Default" w344 {
                  selector: w344 -> [w346 _]
                  tunnel: w341 -> [w347 _]
                  tunnel: w339 -> [w345 _]
                  frame 0, Default {
                    n260 = property class="XYGraph (strict)"(reference=w347, "Active Cursor"=w345, "Cursor.Cursor Plot"=w346) -> ()  [unwired: 1 in, 2 out]
                  }
                  frame -1 {
                  }
                }
              }
              frame Default {
              }
            }
          }
          frame Default {
            n261 = Format Into String(w350, w349, w351, 0 ("input 3")) -> (resulting string=w352:string)  [unwired: 3 in, 1 out]
            n262 = Enqueue Element(queue=w348, element=w352) -> ()  [unwired: 1 in, 4 out]
          }
          frame "DA_CUR_HIDE_1" {
            n263 = Format Into String("DA_CUR_HIDE" ("input 2"), w356, w357, 0 ("input 3")) -> (resulting string=w358:string)  [unwired: 3 in, 1 out]
            n264 = Enqueue Element(queue=w355, element=w358) -> ()  [unwired: 1 in, 4 out]
          }
        }
        n265 = call "CRYPreUpdate Sequence.vi"("EventName"="CurLibUpdate") -> ()  [unwired: 15 in]
      }
      event "PaletteShow": Value Change {
        n266 = event-data() -> ("NewVal"=w360:bool)  [unwired: 6 out]
        n267 = property on="Octave Graph" class="XYGraph (strict)"("Palette Visible"=w360) -> ()  [unwired: 2 in, 2 out]
      }
      event "Cursor": Key Down; "Cursor": Key Repeat {
        n268 = event-data() -> ("ScanCode"=w361:i16)  [unwired: 10 out]
        n269 = case shown="75, 77" w361 {
          selector: w361 -> [_ w377]
          frame 0, Default {
            n270 = local write "DirectionKey"(FALSE ("ScanCode")) -> ()
          }
          frame 75, 77 {
            n271 = local read "NewCursIdx"() -> (w373:u32)
            n272 = property on="Octave Graph" class="XYGraph (strict)"("Active Cursor"=w373) -> (error out=w371:errorcluster, "Cursor.Cursor Plot"=w382:i32, "Value"=w383:cluster{"XY Graph":cluster{dbl, dbl}[]}[])  [unwired: 2 in, 1 out]
            n273 = Index Array(array=w383, index=w382) -> (element=w381:cluster{"XY Graph":cluster{dbl, dbl}[]})
            n274 = property on="Octave Graph" class="XYGraph (strict)"(error in=w371) -> ("Cursor.Cursor X"=w380:dbl)  [unwired: 1 in, 2 out]
            n275 = Unbundle By Name(w381) -> ("XY Graph"=w370:cluster{dbl, dbl}[])
            n276 = for {
              tunnel: w370 -> [w389] mode=indexing
              tunnel: w380 -> [w387]
              tunnel: [w386] -> w369
              i -> [w386]
              stop <- w385 stop-if-true
              n277 = Unbundle(w389) -> (w388:dbl)  [unwired: 1 out]
              n278 = Equal?(x=w388, y=w387) -> (x = y?=w385:bool)
            }
            n279 = Equal?(x=w377, y=i16 77) -> (x = y?=w375:bool)
            n280 = Array Size(array=w370) -> (size(s)=w367:i32)
            n281 = Decrement(x=w367) -> (x-1=w364:i32)
            n282 = Equal?(x=w364, y=w369) -> (x = y?=w368:bool)
            n283 = Increment(x=w369) -> (x+1=w366:i32)
            n284 = Decrement(x=w369) -> (x-1=w374:i32)
            n285 = Select(t=w364, s=w368, f=w366) -> (s? t:f=w365:i32)
            n286 = Select(t=w365, s=w375, f=w374) -> (s? t:f=w372:i32)
            n287 = Index Array(array=w370, index=w372) -> (element=w379:cluster{dbl, dbl})
            n288 = Unbundle(w379) -> (w378:dbl)  [unwired: 1 out]
            n289 = property on="Octave Graph" class="XYGraph (strict)"("Cursor.Cursor X"=w378) -> (error out=w363:errorcluster)  [unwired: 2 in, 1 out]
            n290 = case shown="No Error" w363 {
              frame No Error {
                n291 = property on="CursorPlot" class="Bool (strict)"("Val(Sgnl)"=TRUE ("Value (Signaling)")) -> ()  [unwired: 2 in, 2 out]
              }
              frame Error {
              }
            }
          }
        }
      }
      event "Cursor": Mouse Down {
        n292 = event-data() -> ("CtlRef"=w393:refnum<vi>, "Coords"=w390:T1)  [unwired: 7 out]
        n293 = invoke class="Tbl (strict)" method="Point To Row Column"(reference=w393, "Point"=w390) -> ("CellPosition"=w392:T5)  [unwired: 4 in, 5 out]
        n294 = local write "Cursor Coords"(w390) -> ()
        n295 = Unbundle By Name(w392) -> ("Row"=w391:i32)
        n296 = flat-sequence {
          tunnel: w391 -> [w394]
          frame #0 {
            n297 = Equal To 0?(x=w394) -> (x = 0?=w398:bool)
            n298 = local write "NewCursIdx"(w394) -> ()
            n299 = property on="Octave Graph" class="XYGraph (strict)"("Active Cursor"=w394) -> ()  [unwired: 2 in, 2 out]
            n300 = Select(t=1 ("OldCursIdx"), s=w398, f=0 ("OldCursIdx")) -> (s? t:f=w395:i32)
            n301 = local write "OldCursIdx"(w395) -> ()
          }
          frame #1 {
            n302 = property on="CursorColor" class="Bool (strict)"("Val(Sgnl)"=TRUE ("Value (Signaling)")) -> ()  [unwired: 2 in, 2 out]
          }
        }
      }
      event "Cursor": Value Change {
        n303 = event-data() -> ("OldVal"=w404:string[][], "NewVal"=w403:string[][])  [unwired: 5 out]
        n304 = local read "Cursor Coords"() -> (w401:T1)
        n305 = control-ref of="This VI"() -> (w402:refnum<vi>)
        n306 = call "CRYCursor move in Cursor Table.vi"("NewVal"=w403, "OldVal"=w404, "Cursor Coords"=w401, "pGraph VI"=w402) -> ("NewVal Out"=w400:string[][])  [unwired: 7 in]
        n307 = local write "Cursor"(w400) -> ()
      }
      event "CursorShow": Value Change {
        n308 = event-data() -> ("NewVal"=w405:bool)  [unwired: 6 out]
        n309 = flat-sequence {
          tunnel: w405 -> [w410]
          frame #0 {
            n310 = Select(t="DA_CUR_VIEW", s=w410, f="DA_CUR_HIDE") -> (s? t:f=w409:string)
            n311 = control-ref of="This VI"() -> (w406:refnum<vi>)
            n312 = call "CRYCursor InsDel.vi"("Graph VI Ref"=w406, "sAction"=w409) -> ()  [unwired: 10 in]
          }
          frame #1 {
            n313 = property on="ToolbarUpdate" class="Bool (strict)"("Val(Sgnl)"=TRUE ("Value (Signaling)")) -> ()  [unwired: 2 in, 2 out]
          }
        }
      }
      event "CursorPlot": Value Change {
        n314 = event-data() -> ()  [unwired: 7 out]
        n315 = local read "CursorShow"() -> (w412:bool)
        n316 = case shown="True" w412 {
          frame False {
          }
          frame True {
            n317 = control-ref of="Octave Graph"() -> (w415:refnum<vi>)
            n318 = control-ref of="Cursor"() -> (w414:refnum<vi>)
            n319 = call "CRYPlot Cursor.vi"("Cursor Ref"=w414, "Graph Ref"=w415, "Graph Type"="XY") -> ()  [unwired: 9 in]
          }
        }
      }
      event "CursorColor": Value Change {
        n320 = event-data() -> ()  [unwired: 7 out]
        n321 = local read "NewCursIdx"() -> (w426:u32)
        n322 = local read "OldCursIdx"() -> (w427:u32)
        n323 = property on="Octave Graph" class="XYGraph (strict)"("Active Cursor"=w427) -> ("Cursor.Cursor Color"=w419:u32)  [unwired: 2 in, 2 out]
        n324 = property on="Octave Graph" class="XYGraph (strict)"("Active Cursor"=w426) -> ("Cursor.Cursor Color"=w418:u32)  [unwired: 2 in, 2 out]
        n325 = Bundle By Name(cluster=T5 {"Row"=0, "Column"=0} ("Active Cell:Active Cell"), "Row"=w426, "Column"=0) -> (w423:T5)
        n326 = Bundle By Name(cluster=T5 {"Row"=0, "Column"=0} ("Active Cell:Active Cell"), "Row"=w427, "Column"=0) -> (w420:T5)
        n327 = property on="Cursor" class="Tbl (strict)"("Active Cell"=w420, "CellFontColor"=w419, "Cell BG Color"=u32 16777226) -> ()  [unwired: 2 in, 2 out]
        n328 = property on="Cursor" class="Tbl (strict)"("Active Cell"=w423, "CellFontColor"=w418, "Cell BG Color"=u32 60927) -> ()  [unwired: 2 in, 2 out]
      }
      event "Legend": Mouse Down {
        n329 = event-data() -> ("CtlRef"=w428:refnum<vi>, "Coords"=w434:T1, "Button"=w433:u16)  [unwired: 6 out]
        n330 = local read "TotalPlot"() -> (w430:u32)
        n331 = call "CRYData View Legend Plot OnOff.vi"("TotalPlot"=w430, "Button Info"=w433, "Mouse Point"=w434, "MCListbox Ref In"=w428) -> ("Active Row"=w429:i32, "Visible?"=w431:bool, "Click State"=w432:bool)  [unwired: 5 out]
        n332 = case shown="True" w432 {
          tunnel: w431 -> [_ w447]
          tunnel: w429 -> [_ w448]
          tunnel: w428 -> [_ w442]
          frame False {
          }
          frame True {
            n333 = property class="MCListbox (strict)"(reference=w442) -> ("ItemSyms"=w441:i32[])  [unwired: 1 in, 2 out]
            n334 = property on="Octave Graph" class="XYGraph (strict)"("XScale.ScaleFit"=u8 0 ("Y Scale.Scale Fit")) -> (error out=w444:errorcluster)  [unwired: 2 in, 1 out]
            n335 = property on="AxisChange" class="Bool (strict)"("Val(Sgnl)"=TRUE ("Value (Signaling)")) -> ()  [unwired: 2 in, 2 out]
            n336 = To Unsigned Long Integer(number=w448) -> (unsigned 32bit integer=w446:u32)
            n337 = property on="Octave Graph" class="XYGraph (strict)"(error in=w444, "Active Plot"=w446, "Plot.Visible?"=w447) -> (error out=w436:errorcluster)  [unwired: 1 in, 1 out]
            n338 = for {
              tunnel: w441 -> [w476] mode=indexing
              tunnel: 38 -> [w475]
              shift-right: [w470] -> w437
              shift-left: i32[] [] -> [w471]
              i -> [w473]
              n339 = Equal?(x=w476, y=w475) -> (x = y?=w474:bool)
              n340 = Build Array (concatenate)(w471, w473) -> (w472:i32[])
              n341 = Select(t=w472, s=w474, f=w471) -> (s? t:f=w470:i32[])
            }
            n342 = Array Size(array=w437) -> (size(s)=w438:i32)
            n343 = case shown="1" w438 {
              selector: w438 -> [w452 w462 _]
              tunnel: w437 -> [w451 w461 _]
              tunnel: w436 -> [w450 w459 w469]
              tunnel: [w449 w460 w469] -> w435
              frame 2.. {
                n344 = for {
                  N: w452 -> [_]
                  tunnel: w451 -> [w455] mode=indexing
                  shift-right: [w453] -> w449
                  shift-left: w450 -> [w454]
                  n345 = property on="Octave Graph" class="XYGraph (strict)"(error in=w454, "Active Plot"=w455, "Plot.Plot Interpolation"=u8 3, "Plot.Bar Plot Style"=u8 0, "Plot.Fill To"=i16 -1) -> (error out=w453:errorcluster)  [unwired: 1 in, 1 out]
                }
              }
              frame 1 {
                n346 = for {
                  N: w462 -> [_]
                  tunnel: w461 -> [w465] mode=indexing
                  shift-right: [w464] -> w460
                  shift-left: w459 -> [w463]
                  n347 = property on="Octave Graph" class="XYGraph (strict)"(error in=w463, "Active Plot"=w465, "Plot.Plot Interpolation"=u8 0, "Plot.Bar Plot Style"=u8 2, "Plot.Fill To"=i16 -2) -> (error out=w464:errorcluster)  [unwired: 1 in, 1 out]
                }
              }
              frame Default {
              }
            }
            n348 = case shown="No Error" w435 {
              frame No Error {
              }
              frame Error {
              }
            }
          }
        }
      }
      event "Legend": Double Click {
        n349 = event-data() -> ("CtlRef"=w478:refnum<vi>, "Coords"=w477:T1)  [unwired: 8 out]
        n350 = disable-structure shown="Disabled" {
          disable-tunnel: w478 -> [w484 _]
          disable-tunnel: w477 -> [w483 _]
          frame Disabled {
            n351 = call "CRYGet MultiListBox Click State.vi"("Coords"=w483, "MultiList Box Ref In"=w484) -> ("State"=w482:bool)  [unwired: 6 in, 3 out]
            n352 = call "CRYClick Name in Legend.vi"("Mouse Point"=w483, "MCListbox Ref In"=w484) -> ("Active Row"=w480:i32, "Click State?"=w481:bool)  [unwired: 8 in]
            n353 = And(x=w482, y=w481) -> (x .and. y?=w479:bool)
            n354 = case shown="True" w479 {
              tunnel: w484 -> [_ w485]
              tunnel: w480 -> [_ w486]
              frame False {
              }
              frame True {
                n355 = call "CRYOpen Step by Legend.vi"("Active Row"=w486, "MCListbox Ref In"=w485, "Type"=enum16{"Curves", "Values", "Results", "WFM"}."Curves" ("Type In")) -> ()  [unwired: 9 in]
              }
            }
          }
          frame Enabled {
          }
        }
      }
      event "Legend": Mouse Move {
        n356 = event-data() -> ("CtlRef"=w488:refnum<vi>, "Coords"=w495:T1)  [unwired: 4 out]
        n357 = local read "TotalPlot"() -> (w494:u32)
        n358 = call "CRYData View Legend Mouse Move.vi"("TotalPlot"=w494, "Mouse Point"=w495, "MCListbox Ref In"=w488) -> ("CellSize"=w492:T7, "Position"=w491:T8, "Selected Row"=w490:i32, "Move State"=w489:bool, "CellBG"=w493:u32)  [unwired: 1 in, 3 out]
        n359 = case shown="True" w489 {
          tunnel: w493 -> [_ w501]
          tunnel: w492 -> [_ w500]
          tunnel: w491 -> [_ w499]
          tunnel: w490 -> [_ w498]
          frame False {
            n360 = property on="ColorBox" class="ColBox"("Visible"=FALSE) -> ()  [unwired: 2 in, 2 out]
          }
          frame True {
            n361 = local write "OldRow"(w498) -> ()
            n362 = property on="ColorBox" class="ColBox"("Position"=w499, "Color Area Size"=w500, "Value"=w501, "Visible"=TRUE) -> ()  [unwired: 2 in, 2 out]
          }
        }
      }
      event "Legend": Value Change {
        n363 = event-data() -> ("NewVal"=w502:i32[])  [unwired: 6 out]
        n364 = local read "Test"() -> (w503:string)
        n365 = case shown="Default" w503 {
          tunnel: w502 -> [_ w505]
          frame "Test" {
          }
          frame Default {
            n366 = control-ref of="Legend"() -> (w507:refnum<vi>)
            n367 = local read "GraphType"() -> (w506:string)
            n368 = call "CRYData View Legend Manipulate.vi"("sAction"="GetViewNumbyLegNum", "nData"=w505, "sData"=w506, "Legend Ref"=w507) -> ("nData Out"=w508:i32[])  [unwired: 6 in, 1 out]
            n369 = call "CRYGet Graph Name From Graph Type.vi"("Graph Type"=w506) -> ("Type"=w510:enum16{"Curves", "Values", "Results", "WFM"})  [unwired: 9 in, 1 out]
            n370 = call "CRYTree Global Manipulate.vi"("Type In"=w510) -> ("Tree/Curve Tree"=w509:refnum<vi>)  [unwired: 7 in, 3 out]
            n371 = call "CRYTree Manuplate.vi"("sAction"="SetActiveNumbers", "nData"=w508, "Tree in"=w509) -> ("Tree Out"=w504:refnum<vi>)  [unwired: 5 in, 3 out]
            n372 = flat-sequence {
              tunnel: w504 -> [_]
              frame #0 {
                n373 = call "CRYUpdate Buttons.vi"() -> ()  [unwired: 12 in]
              }
            }
          }
        }
      }
      event "LegendVScrollShow": Value Change {
        w524 = T6 {"Left"=0, "Top"=0, "Right"=0, "Bottom"=0}  # input cluster
        n374 = event-data() -> ("NewVal"=w516:bool)  [unwired: 6 out]
        n375 = property on="Legend" class="MCListbox (strict)"("VScrollVis"=w516) -> ()  [unwired: 2 in, 2 out]
        n376 = control-ref of="PaneLegend"() -> (w514:refnum<vi>)
        n377 = property class="Pane"(reference=w514) -> ("Left"=w523:i32, "Top"=w520:i32, "Width"=w522:u32, "Height"=w519:u32)  [unwired: 1 in, 2 out]
        n378 = Add(x=w523, y=w522) -> (x+y=w521:u32)
        n379 = Add(x=w520, y=w519) -> (x+y=w518:u32)
        n380 = Bundle By Name(cluster=w524, "Left"=w523, "Top"=w520, "Right"=w521, "Bottom"=w518) -> (w517:T6)
        n381 = control-ref of="Legend"() -> (w515:refnum<vi>)
        n382 = local read "LegendVScrollShow"() -> (w513:bool)
        n383 = call "CRYLegend Resize in Graph Window.vi"("VScrollShow"=w513, "Pane Ref"=w514, "input cluster"=w517, "Legend"=w515) -> ()  [unwired: 8 out]
      }
      event "RemoveAll": Value Change {
        w531 = 0 ("Active X Scale")
        w529 = "" ("X Scale.Name Label.Text")
        n384 = event-data() -> ()  [unwired: 7 out]
        n385 = flat-sequence {
          frame #0 {
            n386 = control-ref of="This VI"() -> (w542:refnum<vi>)
            n387 = Build Array(-1 ("nData")) -> (w543:i32[])
            n388 = call "CRYSymbol Conversion.vi"("pGraph VI"=w542, "nDatas"=w543, "sActin"="LEGEND_REMOVE") -> ()  [unwired: 9 in]
          }
          frame #1 {
            n389 = control-ref of="Legend"() -> (w546:refnum<vi>)
            n390 = call "CRYData View Legend Item Delete.vi"("RowNumber"=-1, "Legend MultiListbox In"=w546) -> ()  [unwired: 10 out]
          }
        }
        n391 = local write "TotalPlot"(u32 0 ("TotalPlot")) -> ()
        n392 = local write "OldRow"(-1 ("OldRow 2")) -> ()
        n393 = local read "CursorShow"() -> (w526:bool)
        n394 = local write "CursorEnabled"(FALSE ("CursorEnabled")) -> ()
        n395 = case shown="True" w526 {
          tunnel: w525 -> [_ w537]
          frame False {
          }
          frame True {
            n396 = local read "Graph Number"() -> (w535:i32)
            n397 = Format Into String("DA_CUR_HIDE" ("input 1"), "AAA" ("input 2"), w535, 0 ("input 3")) -> (resulting string=w539:string)  [unwired: 3 in, 1 out]
            n398 = Enqueue Element(queue=w537, element=w539) -> ()  [unwired: 1 in, 4 out]
          }
        }
        n399 = local write "Octave Graph"(cluster{"XY Graph":cluster{dbl, dbl}[]}[] [] ("XY Graph")) -> ()
        n400 = property on="Octave Graph" class="XYGraph (strict)"("ActXScl"=w531, "XScale.NameLbl.Text"=w529, "ActYScl"=w531, "YScale.NameLbl.Text"=w529, "ActYScl"=1 ("Active Y Scale"), "YScale.NameLbl.Text"=w529, "YScale.Visible"=FALSE ("Y Scale.Visible")) -> ()  [unwired: 2 in, 2 out]
      }
      event "RemoveSome": Value Change {
        n401 = event-data() -> ()  [unwired: 7 out]
        n402 = flat-sequence {
          tunnel: [w550] -> w548
          tunnel: [w557] -> w547
          tunnel: w548 -> [w581]
          tunnel: w547 -> [w580]
          frame #0 {
            n403 = local read "SelectedRow"() -> (w556:i32[])
            n404 = control-ref of="Legend"() -> (w552:refnum<vi>)
            n405 = local read "GraphType"() -> (w551:string)
            n406 = Reverse 1D Array(array=w556) -> (reversed array=w550:i32[])
            n407 = for {
              shift-right: [w560] -> w557
              shift-left: _ -> [w559]
              tunnel: w550 -> [w558] mode=indexing
              n408 = local read "TotalPlot"() -> (w564:u32)
              n409 = Decrement(x=w564) -> (x-1=w561:u32)
              n410 = Increment(x=w558) -> (x+1=w563:i32)
              n411 = Subtract(x=w561, y=w558) -> (x-y=w562:u32)
              n412 = for {
                N: w562 -> [_]
                tunnel: w563 -> [w579]
                shift-right: [w567] -> w560
                shift-left: w559 -> [w566]
                i -> [w578]
                n413 = Add(x=w579, y=w578) -> (x+y=w576:i32)
                n414 = property on="Octave Graph" class="XYGraph (strict)"(error in=w566, "Active Plot"=w576) -> (error out=w565:errorcluster, "Plot.Plot Color"=w575:u32, "Plot.Fill/Pt. Color"=w574:u32, "Plot.Line Style"=w573:u8, "Plot.Line Width"=w572:u8, "Plot.Point Style"=w571:u8, "Plot.Plot Interpolation"=w570:u8, "Plot.Bar Plot Style"=w569:u8, "Plot.Fill To"=w568:i16)  [unwired: 1 in, 1 out]
                n415 = Decrement(x=w576) -> (x-1=w577:i32)
                n416 = property on="Octave Graph" class="XYGraph (strict)"(error in=w565, "Active Plot"=w577, "Plot.Plot Color"=w575, "Plot.Fill/Pt. Color"=w574, "Plot.Line Style"=w573, "Plot.Line Width"=w572, "Plot.Point Style"=w571, "Plot.Plot Interpolation"=w570, "Plot.Bar Plot Style"=w569, "Plot.Fill To"=w568) -> (error out=w567:errorcluster)  [unwired: 1 in, 1 out]
              }
              n417 = local write "TotalPlot"(w561) -> ()
            }
            n418 = call "CRYData View Legend Manipulate.vi"("sAction"="GetGlobalNumbyLegNum", "nData"=w550, "sData"=w551, "Legend Ref"=w552) -> ("nData Out"=w549:i32[])  [unwired: 6 in, 1 out]
            n419 = control-ref of="This VI"() -> (w554:refnum<vi>)
            n420 = call "CRYSymbol Conversion.vi"("pGraph VI"=w554, "nDatas"=w549, "sActin"="LEGEND_REMOVE") -> ()  [unwired: 9 in]
          }
          frame #1 {
            n421 = for {
              tunnel: w581 -> [w582] mode=indexing
              n422 = local read "Octave Graph"() -> (w584:cluster{"XY Graph":cluster{dbl, dbl}[]}[])
              n423 = control-ref of="Legend"() -> (w585:refnum<vi>)
              n424 = Delete From Array(array=w584, index=w582) -> (array with subset deleted=w583:cluster{"XY Graph":cluster{dbl, dbl}[]}[])  [unwired: 1 in, 1 out]
              n425 = local write "Octave Graph"(w583) -> ()
              n426 = call "CRYData View Legend Item Delete.vi"("RowNumber"=w582, "Legend MultiListbox In"=w585) -> ()  [unwired: 10 out]
            }
            n427 = case shown="No Error" w580 {
              frame No Error {
              }
              frame Error {
              }
            }
          }
          frame #2 {
            n428 = local read "TotalPlot"() -> (w586:u32)
            n429 = case shown="1, Default" w586 {
              selector: w586 -> [_ w618]
              frame 0 {
                n430 = property on="RemoveAll" class="Bool (strict)"("Val(Sgnl)"=TRUE ("Value (Signaling)")) -> ()  [unwired: 2 in, 2 out]
              }
              frame 1, Default {
                n431 = for {
                  N: w618 -> [_]
                  tunnel: [w619] -> w617
                  i -> [w622]
                  n432 = property on="Legend" class="MCListbox (strict)"() -> ("ItemSyms"=w625:i32[])  [unwired: 2 in, 2 out]
                  n433 = Bundle By Name(cluster=T5 {"Row"=0, "Column"=0} ("Active Cell:Active Cell"), "Row"=w622, "Column"=1) -> (w626:T5)
                  n434 = Index Array(array=w625, index=w622) -> (element=w623:i32)
                  n435 = property on="Legend" class="MCListbox (strict)"("ActiveCell"=w626) -> ("CellBG"=w621:u32)  [unwired: 2 in, 2 out]
                  n436 = Equal?(x=w623, y=38) -> (x = y?=w620:bool)
                  n437 = property on="Octave Graph" class="XYGraph (strict)"("Active Plot"=w622, "Plot.Plot Color"=w621, "Plot.Fill/Pt. Color"=w621, "Plot.Visible?"=w620) -> (error out=w619:errorcluster)  [unwired: 2 in, 1 out]
                }
                n438 = case shown="No Error" w617 {
                  frame No Error {
                  }
                  frame Error {
                  }
                }
              }
            }
            n439 = case shown="2.." w586 {
              selector: w586 -> [w589 w603 _]
              frame 2.. {
                n440 = for {
                  N: w589 -> [_]
                  shift-right: [w592] -> w588
                  shift-left: _ -> [w591]
                  i -> [w593]
                  n441 = property on="Octave Graph" class="XYGraph (strict)" props=["Active Plot", "Plot", "Plot Color", "Plot", "Fill/Pt. Color", "Plot", "Line Style", "Plot", "Line Width", "Plot", "Point Style", "Plot", "Plot Interpolation", "Plot", "Bar Plot Style", "Plot", "Fill To"](error in=w591, "Active Plot"=w593) -> (error out=w590:errorcluster, "Plot.Plot Color"=w601:u32, "Plot.Fill/Pt. Color"=w600:u32, "Plot.Line Style"=w599:u8, "Plot.Line Width"=w598:u8, "Plot.Point Style"=w597:u8)  [unwired: 1 in, 4 out]
                  n442 = property on="Octave Graph" class="XYGraph (strict)"(error in=w590, "Active Plot"=w593, "Plot.Plot Color"=w601, "Plot.Fill/Pt. Color"=w600, "Plot.Line Style"=w599, "Plot.Line Width"=w598, "Plot.Point Style"=w597, "Plot.Plot Interpolation"=u8 3, "Plot.Bar Plot Style"=u8 0, "Plot.Fill To"=i16 -1) -> (error out=w592:errorcluster)  [unwired: 1 in, 1 out]
                }
                n443 = case shown="No Error" w588 {
                  frame No Error {
                  }
                  frame Error {
                  }
                }
              }
              frame 1 {
                n444 = for {
                  N: w603 -> [_]
                  shift-right: [w606] -> w602
                  shift-left: _ -> [w605]
                  i -> [w610]
                  n445 = property on="Octave Graph" class="XYGraph (strict)" props=["Active Plot", "Plot", "Plot Color", "Plot", "Fill/Pt. Color", "Plot", "Line Style", "Plot", "Line Width", "Plot", "Point Style", "Plot", "Plot Interpolation", "Plot", "Bar Plot Style", "Plot", "Fill To"](error in=w605, "Active Plot"=w610) -> (error out=w604:errorcluster, "Plot.Plot Color"=w615:u32, "Plot.Fill/Pt. Color"=w614:u32, "Plot.Line Style"=w613:u8, "Plot.Line Width"=w612:u8, "Plot.Point Style"=w611:u8)  [unwired: 1 in, 4 out]
                  n446 = property on="Octave Graph" class="XYGraph (strict)"(error in=w604, "Active Plot"=w610, "Plot.Plot Color"=w615, "Plot.Fill/Pt. Color"=w614, "Plot.Line Style"=w613, "Plot.Line Width"=w612, "Plot.Point Style"=w611, "Plot.Plot Interpolation"=u8 0, "Plot.Bar Plot Style"=u8 2, "Plot.Fill To"=i16 -2) -> (error out=w606:errorcluster)  [unwired: 1 in, 1 out]
                }
                n447 = case shown="No Error" w602 {
                  frame No Error {
                  }
                  frame Error {
                  }
                }
              }
              frame Default {
              }
            }
            n448 = property on="AxisChange" class="Bool (strict)"("Val(Sgnl)"=TRUE ("Value (Signaling)")) -> ()  [unwired: 2 in, 2 out]
          }
        }
      }
      event "AxisChange": Value Change {
        w644 = enum16{"Curves", "Values", "Results", "WFM"}."Curves" ("Type In")
        n449 = event-data() -> ()  [unwired: 7 out]
        n450 = control-ref of="Legend"() -> (w645:refnum<vi>)
        n451 = call "CRYGet Graph Data in Graph.vi"("Graph Type"="XY", "Legend Refnum"=w645, "Type In"=w644) -> ("Rows"=w636:i32[])  [unwired: 4 in, 4 out]
        n452 = property on="Legend" class="MCListbox (strict)"() -> ("ItemSyms"=w646:i32[])  [unwired: 2 in, 2 out]
        n453 = for {
          tunnel: w646 -> [w654] mode=indexing
          shift-right: [w653] -> w637
          shift-left: i32[] [] -> [w652]
          tunnel: w636 -> [w651] mode=indexing
          shift-right: [w648] -> w643
          shift-left: i32[] [] -> [w647]
          i -> [w649]
          n454 = Equal?(x=38, y=w654) -> (x = y?=w650:bool)
          n455 = case shown="True" w650 {
            tunnel: [w657 w663] -> w653
            tunnel: w652 -> [w657 w662]
            tunnel: w651 -> [_ w661]
            tunnel: w649 -> [_ w660]
            tunnel: [w656 w659] -> w648
            tunnel: w647 -> [w656 w658]
            frame False {
            }
            frame True {
              n456 = Insert Into Array(array=w658, new element=w660) -> (w659:i32[])  [unwired: 1 in]
              n457 = Insert Into Array(array=w662, new element=w661) -> (w663:i32[])  [unwired: 1 in]
            }
          }
        }
        n458 = call "CRYGet Legend Name.vi"("MCListbox Refnum"=w645) -> ("Names Out"=w639:string[])  [unwired: 10 in]
        n459 = control-ref of="This VI"() -> (w629:refnum<vi>)
        n460 = for {
          tunnel: w639 -> [w669]
          tunnel: w643 -> [w670] mode=indexing
          tunnel: [w666] -> w642 mode=indexing
          tunnel: [w665] -> w640
          tunnel: w644 -> [w664]
          n461 = Index Array(array=w669, index=w670) -> (element=w668:string)
          n462 = call "CRYGet Curve Library Data.vi"("Type"=w664, "Data Name"=w668) -> ("Curve"=w667:T9)  [unwired: 4 out]
          n463 = Unbundle By Name(w667) -> ("Y unit"=w666:string, "X unit"=w665:string)
        }
        n464 = call "CRYGet Two Units Rows.vi"("pGraph VI In"=w629, "Old Rows In"=w637, "Type"=w644) -> ("Unit2"=w633:string, "Unit1"=w641:string, "Two Units"=w632:i32)  [unwired: 2 in, 4 out]
        n465 = case shown="0" w632 {
          selector: w632 -> [w680 w688 w693]
          tunnel: w641 -> [w683 _ w698]
          tunnel: w633 -> [w685 _ _]
          tunnel: w640 -> [w681 _ w696]
          tunnel: [w680 w688 w693] -> w631
          frame 2, Default {
            n466 = property on="Octave Graph" class="XYGraph (strict)"("ActXScl"=0 ("Active X Scale"), "XScale.NameLbl.Text"=w681, "ActYScl"=0 ("Active Y Scale"), "YScale.NameLbl.Text"=w683, "ActYScl"=1 ("Active Y Scale"), "YScale.Visible"=TRUE ("Y Scale.Visible"), "YScale.NameLbl.Text"=w685) -> ()  [unwired: 2 in, 2 out]
          }
          frame 0 {
            w692 = 0 ("Active X Scale")
            w690 = "" ("X Scale.Name Label.Text")
            n467 = property on="Octave Graph" class="XYGraph (strict)"("ActXScl"=w692, "XScale.NameLbl.Text"=w690, "ActYScl"=w692, "YScale.NameLbl.Text"=w690, "ActYScl"=1 ("Active Y Scale"), "YScale.NameLbl.Text"=w690, "YScale.Visible"=FALSE ("Y Scale.Visible")) -> ()  [unwired: 2 in, 2 out]
          }
          frame 1 {
            n468 = property on="Octave Graph" class="XYGraph (strict)"("ActXScl"=0 ("Active X Scale"), "XScale.NameLbl.Text"=w696, "ActYScl"=0 ("Active Y Scale"), "YScale.NameLbl.Text"=w698, "ActYScl"=1 ("Active Y Scale"), "YScale.Visible"=FALSE ("Y Scale.Visible")) -> ()  [unwired: 2 in, 2 out]
          }
        }
        n469 = for {
          tunnel: w643 -> [w679] mode=indexing
          tunnel: w642 -> [w677] mode=indexing
          tunnel: w641 -> [w678]
          shift-right: [w672] -> w630
          shift-left: _ -> [w671]
          n470 = Equal?(x=w678, y=w677) -> (x = y?=w676:bool)
          n471 = Select(t=u32 0 ("Plot.Y Scale Index"), s=w676, f=u32 1 ("Plot.Y Scale Index")) -> (s? t:f=w673:u32)
          n472 = property on="Octave Graph" class="XYGraph (strict)"(error in=w671, "Active Plot"=w679, "Plot.YScaleIdx"=w673) -> (error out=w672:errorcluster)  [unwired: 1 in, 1 out]
        }
        n473 = property on="Repaint Watermark" class="DigNum (strict)"("Val(Sgnl)"=w631) -> ()  [unwired: 2 in, 2 out]
        n474 = case shown="No Error" w630 {
          frame No Error {
          }
          frame Error {
          }
        }
      }
      event "ColorBox": Value Change {
        # "Graph Color Changing"
        n475 = event-data() -> ("NewVal"=w702:u32)  [unwired: 6 out]
        n476 = local read "OldRow"() -> (w703:i32)
        n477 = local read "Event Name"() -> (w700:string)
        n478 = flat-sequence {
          tunnel: [w713] -> w704
          tunnel: w702 -> [w713]
          tunnel: w703 -> [w712]
          tunnel: w704 -> [w714]
          frame #0 {
            n479 = To Unsigned Long Integer(number=w712) -> (unsigned 32bit integer=w711:u32)
            n480 = property on="Legend" class="MCListbox (strict)"("CellBG"=w713) -> ()  [unwired: 2 in, 2 out]
            n481 = property on="Octave Graph" class="XYGraph (strict)"("Active Plot"=w711) -> (error out=w710:errorcluster)  [unwired: 2 in, 1 out]
            n482 = case shown="No Error" w710 {
              frame No Error {
              }
              frame Error {
              }
            }
          }
          frame #1 {
            n483 = property on="Octave Graph" class="XYGraph (strict)"("Plot.Plot Color"=w714) -> ()  [unwired: 2 in, 2 out]
            n484 = property on="ColorBox" class="ColBox"("Visible"=FALSE) -> ()  [unwired: 2 in, 2 out]
          }
        }
        n485 = call "CRYPreUpdate Sequence.vi"("EventName"="CurLibUpdate") -> ()  [unwired: 15 in]
        n486 = case shown="Default" w700 {
          tunnel: w703 -> [_ w708]
          tunnel: w702 -> [_ w707]
          frame "ViewReport" {
          }
          frame Default {
            n487 = control-ref of="Legend"() -> (w706:refnum<vi>)
            n488 = call "CRYSet Plot Settings.vi"("sAction"="Color", "Color"=w707, "Row"=w708, "Legend Refnum"=w706, "Type"=enum16{"Curves", "Values", "Results", "WFM"}."Curves") -> ()  [unwired: 2 in, 5 out]
          }
        }
      }
      event "ColorBox": Mouse Down {
        n489 = event-data() -> ()  [unwired: 9 out]
        n490 = local read "OldRow"() -> (w719:i32)
        n491 = Bundle By Name(cluster=T5 {"Row"=0, "Column"=0} ("Active Cell:Active Cell"), "Row"=w719, "Column"=1) -> (w716:T5)
        n492 = property on="Legend" class="MCListbox (strict)"("ActiveCell"=w716) -> ()  [unwired: 2 in, 2 out]
      }
      event "Octave Graph": Drag Enter {
        n493 = event-data() -> ("Available Data Names"=w720:string[])  [unwired: 1 out]
        n494 = disable-structure shown="Disabled" {
          disable-tunnel: [w723 TRUE] -> w721
          disable-tunnel: w720 -> [w722 _]
          frame Disabled {
            n495 = Search 1D Array(1D array=w722, element="CRY_GRAPH_DATA") -> (index of element=w725:i32)  [unwired: 1 out]
            n496 = Not Equal?(x=w725, y=-1) -> (x != y?=w723:bool)
          }
          frame Enabled {
          }
        }
        n497 = event-data("Accepted?"=w721) -> ()  [unwired: 1 in, 1 out]
      }
      event "Octave Graph": Drop {
        n498 = event-data() -> ()  [unwired: 2 out]
        n499 = local read "Event Name"() -> (w728:string)
        n500 = local read "TotalPlot"() -> (w729:u32)
        n501 = control-ref of="This VI"() -> (w730:refnum<vi>)
        n502 = call "CRYDrop Data in Same Graph.vi"("pGraph VI"=w730, "Queue"=w731, "Total Plot In"=w729, "sAction"=w728) -> ("Accepted?"=w732:bool, "Total Plot Out"=w733:u32)  [unwired: 3 in, 3 out]
        n503 = local write "TotalPlot"(w733) -> ()
        n504 = event-data("Accepted?"=w732) -> ()  [unwired: 1 in, 1 out]
      }
      event "Octave Graph": Cursor Grab {
        n505 = event-data() -> ("CursIdx"=w734:i32)  [unwired: 1 out]
        n506 = flat-sequence {
          tunnel: w734 -> [w735]
          frame #0 {
            n507 = Equal To 0?(x=w735) -> (x = 0?=w736:bool)
            n508 = local write "NewCursIdx"(w735) -> ()
            n509 = Select(t=u32 1 ("OldCursIdx"), s=w736, f=u32 0 ("OldCursIdx")) -> (s? t:f=w739:u32)
            n510 = local write "OldCursIdx"(w739) -> ()
          }
          frame #1 {
            n511 = property on="CursorColor" class="Bool (strict)"("Val(Sgnl)"=TRUE ("Value (Signaling)")) -> ()  [unwired: 2 in, 2 out]
          }
        }
      }
      event "Octave Graph": Cursor Move {
        n512 = event-data() -> ()  [unwired: 10 out]
        n513 = property on="CursorPlot" class="Bool (strict)"("Val(Sgnl)"=TRUE ("Value (Signaling)")) -> ()  [unwired: 2 in, 2 out]
      }
      event "ReportDrop": Value Change {
        n514 = event-data() -> ()  [unwired: 7 out]
        n515 = local read "Event Name"() -> (w742:string)
        n516 = local read "TotalPlot"() -> (w746:u32)
        n517 = control-ref of="This VI"() -> (w744:refnum<vi>)
        n518 = call "CRYDrop Data in Same Graph.vi"("pGraph VI"=w744, "Queue"=w743, "Total Plot In"=w746, "sAction"=w742) -> ("Total Plot Out"=w745:u32)  [unwired: 3 in, 4 out]
        n519 = local write "TotalPlot"(w745) -> ()
      }
      event "Octave Graph": Scale Range Change {
        n520 = event-data() -> ("Kind"=w747:enum16{"X-Scale", "Y-Scale", "Z-Scale"})  [unwired: 8 out]
        n521 = case shown="\"X-Scale\", Default" w747 {
          frame "X-Scale", Default {
            n522 = property on="Octave Graph" class="XYGraph (strict)"("XScale.ScaleFit"=u8 0 ("X Scale.Scale Fit")) -> ()  [unwired: 2 in, 2 out]
          }
          frame "Y-Scale" {
            n523 = property on="Octave Graph" class="XYGraph (strict)"("YScale.ScaleFit"=u8 0 ("Y Scale.Scale Fit")) -> ()  [unwired: 2 in, 2 out]
            n524 = property on="Repaint Watermark" class="DigNum (strict)"("Val(Sgnl)"=-1 ("Value (Signaling)")) -> ()  [unwired: 2 in, 2 out]
          }
        }
      }
      event "Repaint Watermark": Value Change {
        # "Repaint Watermark: 0-none, 1-Unit 1, 2-Unit 1 & 2, -1: surely replot"
        n525 = event-data() -> ("OldVal"=w756:i32, "NewVal"=w752:i32)  [unwired: 5 out]
        n526 = Equal?(x=-1 ("y"), y=w752) -> (x = y?=w753:bool)
        n527 = case shown="False" w753 {
          tunnel: w756 -> [w759 w774]
          tunnel: w752 -> [w757 _]
          tunnel: [w758 "Replot" ("PropertyTab")] -> w754
          tunnel: [w757 w774] -> w751
          frame False {
            n528 = Not Equal?(x=w759, y=w757) -> (x != y?=w760:bool)
            n529 = case shown="True" w760 {
              tunnel: w759 -> [_ w767]
              tunnel: w757 -> [_ w766]
              tunnel: [_ w761] -> w758
              frame False {
              }
              frame True {
                n530 = Equal To 0?(x=w767) -> (x = 0?=w771:bool)
                n531 = Equal?(x=w766, y=1) -> (x = y?=w772:bool)
                n532 = Equal?(x=w767, y=1) -> (x = y?=w765:bool)
                n533 = Equal To 0?(x=w766) -> (x = 0?=w764:bool)
                n534 = And(x=w765, y=w764) -> (x .and. y?=w763:bool)
                n535 = And(x=w771, y=w772) -> (x .and. y?=w769:bool)
                n536 = Or(x=w769, y=w763) -> (x .or. y?=w762:bool)
                n537 = case shown="False" w762 {
                  tunnel: ["Replot" ("PropertyTab") _] -> w761
                  frame False {
                  }
                  frame True {
                  }
                }
              }
            }
          }
          frame True {
          }
        }
        n538 = case shown="\"Replot\"" w754 {
          frame Default {
          }
          frame "Replot" {
            n539 = local read "Event Name"() -> (w776:string)
            n540 = control-ref of="Octave Graph"() -> (w777:refnum<vi>)
            n541 = call "CRYPaint WaterMark.vi"("Type"=w776, "Graph Ref"=w777) -> ()  [unwired: 10 in]
          }
        }
        n542 = local write "Repaint Watermark"(w751) -> ()
      }
      event "OpenProperty": Value Change {
        n543 = event-data() -> ()  [unwired: 7 out]
        n544 = flat-sequence {
          frame #0 {
            n545 = local read "PropertyTab"() -> (w778:string)
            n546 = control-ref of="This VI"() -> (w779:refnum<vi>)
            n547 = call "CRYGraph Property Window Main.vi"("TabName"=w778, "pGraph VI In"=w779) -> ()  [unwired: 1 in, 9 out]
          }
          frame #1 {
            n548 = local write "PropertyTab"("" ("PropertyTab")) -> ()
          }
        }
      }
      event "ToolbarUpdate": Value Change {
        n549 = event-data() -> ()  [unwired: 7 out]
        n550 = local read "Test"() -> (w781:string)
        n551 = case shown="Default" w781 {
          frame Default {
            n552 = local read "Event Name"() -> (w782:string)
            n553 = case shown="Default" w782 {
              frame "ViewReport" {
              }
              frame Default {
                n554 = control-ref of="This VI"() -> (w784:refnum<vi>)
                n555 = call "CRYUpdate DataView Toolbar.vi"("pVI"=w784) -> ()  [unwired: 11 in]
                n556 = call "CRYPreUpdate Sequence.vi"("EventName"="CurLibUpdate") -> ()  [unwired: 15 in]
              }
            }
          }
          frame "Test" {
          }
        }
      }
    }
    n557 = global read "CRYMain Sub Window Global.vi" "gStop"() -> (w82:bool)
    n558 = Or(x=w82, y="stop") -> (x .or. y?=w78:bool)
  }
  n559 = flat-sequence {
    tunnel: w1 -> [_]
    frame #0 {
      n560 = local write "StateOut"(TRUE ("StateOut")) -> ()
    }
  }
